vi "添加启动项.vi"(8 "error in (no error)":errorcluster caption="错误输入（无错误）") -> (0 "error out":errorcluster caption="错误输出", 3 "添加成功标记":bool)   [LabVIEW 2016]
uses:
  <vilib>/registry/registry.llb/Registry RtKey.ctl
  <vilib>/registry/registry.llb/Write Registry Value Simple STR.vi
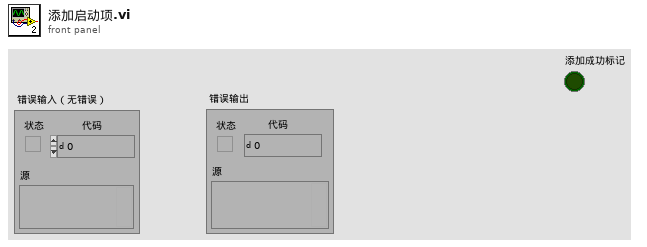
[diagram p1: front panel]
types:
  T1 = typedef "Registry RtKey.ctl" = enum32{"HKEY_CLASSES_ROOT", "HKEY_CURRENT_USER", "HKEY_LOCAL_MACHINE", "HKEY_USERS", "HKEY_PERFORMANCE_DATA", "HKEY_CURRENT_CONFIG", "HKEY_DYN_DATA"}
  T2 = typedef "Registry refnum.ctl" = refnum<k1>
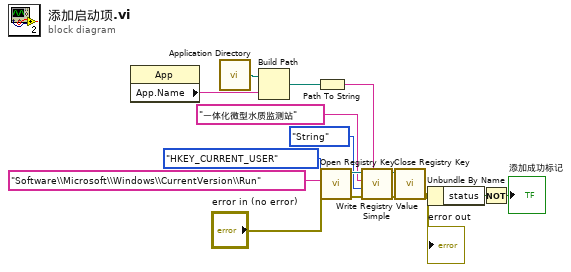
[diagram p0: block diagram]
diagram:
  n1 = property class="App"() -> ("App.Name"=w15:string)  [unwired: 2 in, 2 out]
  n2 = call <vilib>:"Application Directory.vi"() -> ("Application Directory"=w16:path)
  n3 = Build Path(base path=w16, name or relative path=w15) -> (appended path=w1:path)
  n4 = Path To String(path=w1) -> (string=w3:string)
  n5 = call <vilib>:"Open Registry Key.vi"("error in (no error)"="error in (no error)", "subkey"="Software\\Microsoft\\Windows\\CurrentVersion\\Run", "root key (HKEY_LOCAL_MACHINE)"=Registry_RtKey."HKEY_CURRENT_USER") -> ("error out"=w11:errorcluster, "refnum out"=w10:T2)  [unwired: 7 in]
  n6 = call-poly <vilib>:"Write Registry Value Simple.vi"("String/Binary data"=w3, "error in (no error)"=w11, "simple data type"=enum16{"String", "Binary", "DWORD"}."String", "value"="一体化微型水质监测站", "refnum"=w10) -> ("error out"=w13:errorcluster, "refnum out"=w12:T2)  [unwired: 3 in]
  n7 = call <vilib>:"Close Registry Key.vi"("error in (no error)"=w13, "refnum"=w12) -> ("error out"=w5:errorcluster)  [unwired: 5 in]
  "error out" <- w5
  n8 = Unbundle By Name(w5) -> ("status"=w4:bool)
  n9 = Not(x=w4) -> (.not. x?=→"添加成功标记":bool)
